vi "Get error details.vi"(8 "error in (no error)":errorcluster, 11 "JSONMessage in":refnum<class "WampMessage JSON.lvclass">) -> (0 "error out":errorcluster, 2 "Combined Error (JSON)":T1={"Error?"=FALSE, "WAMP Error"={"URI"="", "Arguments Payload"="", "ArgumentKw Payload"="{}", "Details"="{}", "Associated LabVIEW Error"={"status"=FALSE, "code"=0, "source"=""}}, "Associated LabVIEW Error"={"status"=FALSE, "code"=0, "source"=""}}, 3 "JSONMessage out":refnum<class "WampMessage JSON.lvclass">)   [LabVIEW 2020]
uses:
  WAMP Client/API/TypeDefs/Error or abort detail (JSON).ctl
  wamplv.lvlib
  <vilib>/Utility/error.llb/Error Cluster From Error Code.vi
  <vilib>/ErrorRing/Error Ring.xnode
  WampMessage JSON.lvclass
  WAMP Client/API/TypeDefs/Combined error.ctl
  Utils/Utils.lvclass
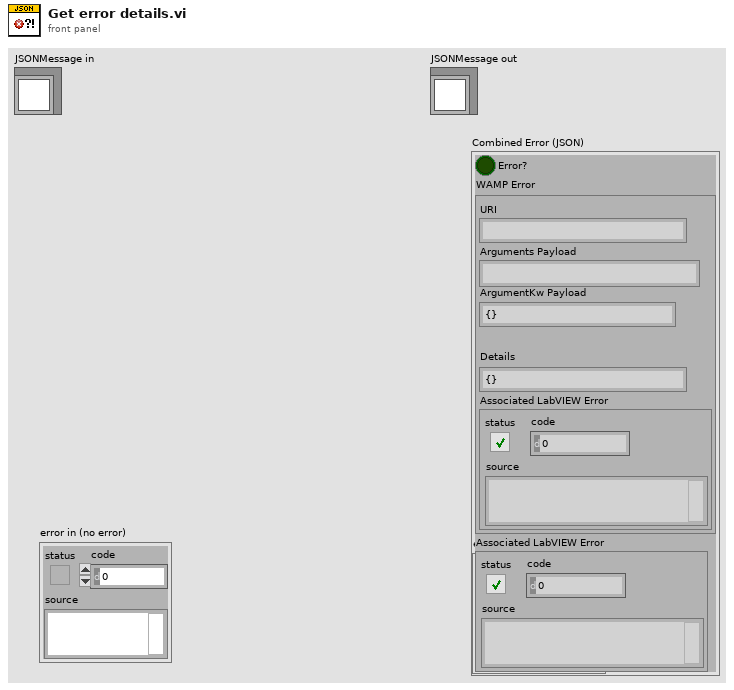
[diagram p1: front panel]
types:
  T1 = typedef "wamplv.lvlib/Combined error.ctl" = cluster{"Error?":bool, "WAMP Error":T2, "Associated LabVIEW Error":errorcluster}
  T2 = typedef "wamplv.lvlib/Error or abort detail (JSON).ctl" = cluster{"URI":string, "Arguments Payload":string, "ArgumentKw Payload":string, "Details":string, "Associated LabVIEW Error":errorcluster}
  T3 = typedef "wamplv.lvlib/WAMP Message Codes.ctl" = enum8{"HELLO", "WELCOME", "CHALLENGE", "AUTHENTICATE", "ABORT", "GOODBYE", "ERROR", "PUBLISH", "PUBLISHED", "SUBSCRIBE", "SUBSCRIBED", "UNSUBSCRIBE", "UNSUBSCRIBED", "EVENT", "CALL", "RESULT", "REGISTER", "REGISTERED", "UNREGISTER", "UNREGISTERED", "INVOCATION", "YIELD"}
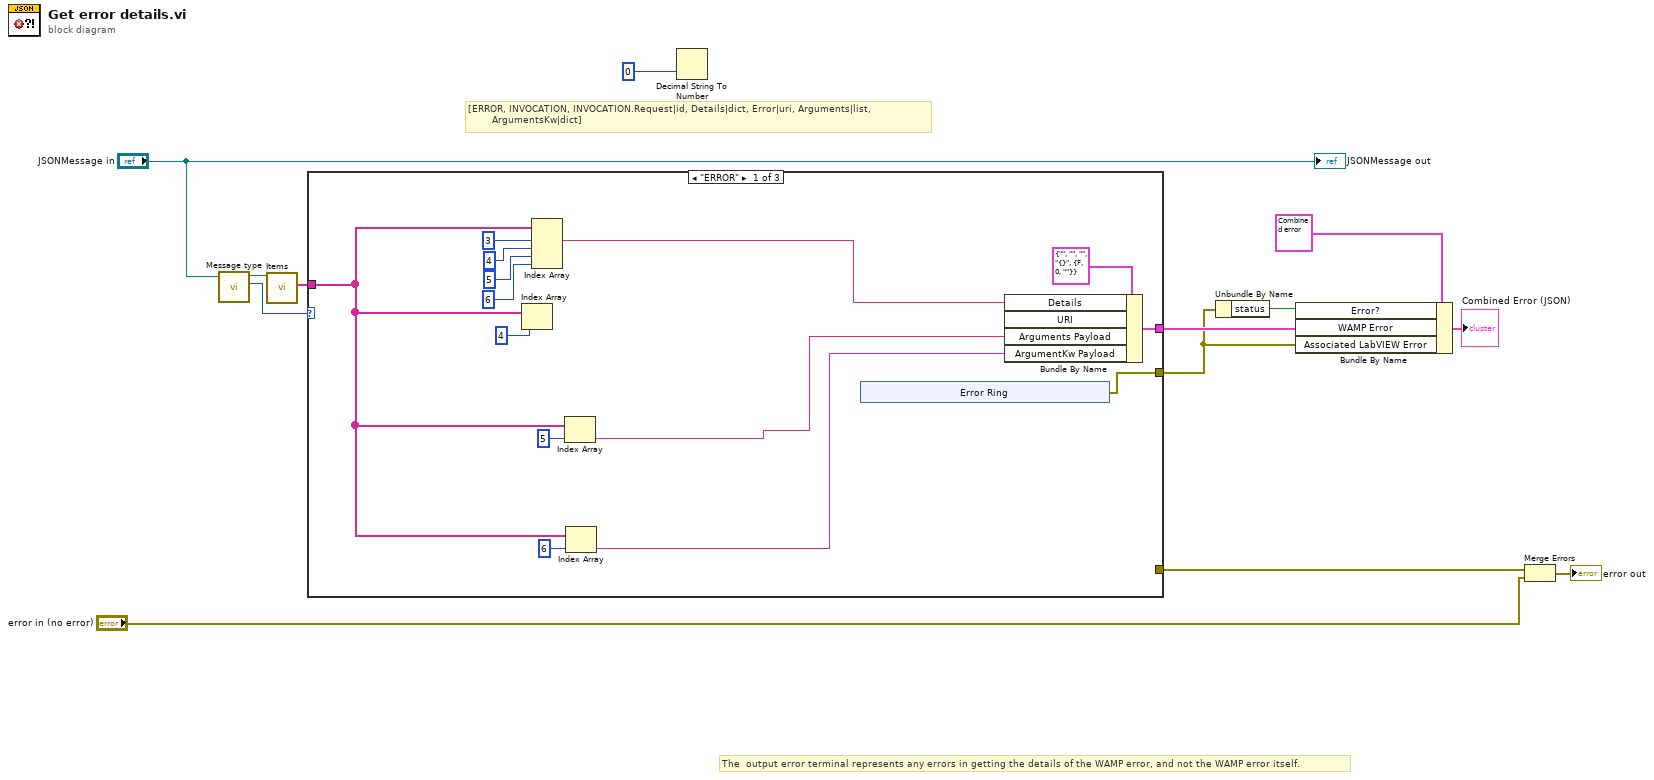
[diagram p0: block diagram]
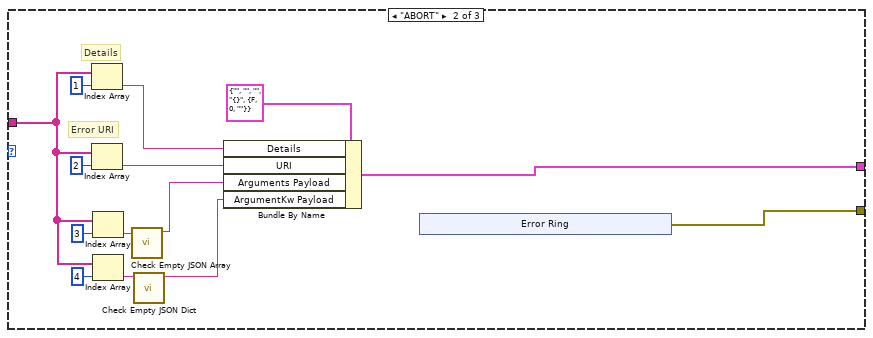
[diagram p2: hidden frame]
diagram:
  # "[ERROR, INVOCATION, INVOCATION.Request|id, Details|dict, Error|uri, Arguments|list,\n        ArgumentsKw|dict]"
  # "The  output error terminal represents any errors in getting the details of the WAMP error, and not the WAMP error itself."
  n1 = call-dynamic "Message type.vi"("JSONMessage in"="JSONMessage in") -> ("Message Codes"=w12:T3, "JSONMessage out"=w13:refnum<class "WampMessage JSON.lvclass">)  [unwired: 9 in]
  n2 = call-dynamic "Items.vi"("JSONMessage in"=w13) -> ("<JSON>Elements"=w11:string[])  [unwired: 9 in, 1 out]
  n3 = case shown="\"ERROR\"" w12 {
    tunnel: w11 -> [w28 w35 _]
    tunnel: [w23 w41 _] -> w7
    tunnel: [w24 w40 _] -> w8
    tunnel: [_ _ _] -> w6
    frame "ERROR" {
      # "ERROR"
      n4 = Index Array(array=w28, index=4) -> ()  [unwired: 1 out]
      n5 = Index Array(array=w28, index #1=3 ("index"), index #2=4 ("index"), index #3=5 ("index"), index #4=6 ("index")) -> (element #1=w21:string)  [unwired: 3 out]
      n6 = Index Array(array=w28, index=5) -> (element=w25:string)
      n7 = Index Array(array=w28, index=6) -> (element=w26:string)
      n8 = xnode "Error Ring"() -> ("error out"=w23:errorcluster)
      n9 = Bundle By Name(cluster=T2 {"URI"="", "Arguments Payload"="", "ArgumentKw Payload"="", "Details"="{}", "Associated LabVIEW Error"={"status"=FALSE, "code"=0, "source"=""}} ("Cluster"), "Details"=w21, "Arguments Payload"=w25, "ArgumentKw Payload"=w26) -> (w24:T2)  [unwired: 1 in]
    }
    frame "ABORT" {
      # "Details"
      # "Error URI"
      # "ABORT"
      n10 = Index Array(array=w35, index=1) -> (element=w44:string)
      n11 = Index Array(array=w35, index=2) -> (element=w45:string)
      n12 = Index Array(array=w35, index=3) -> (element=w37:string)
      n13 = Index Array(array=w35, index=4) -> (element=w36:string)
      n14 = call "Check Empty JSON Array.vi"("JSON in"=w37) -> ("JSON out"=w34:string)  [unwired: 10 in]
      n15 = call "Check Empty JSON Dict.vi"("JSON in"=w36) -> ("JSON out"=w33:string)  [unwired: 10 in]
      n16 = Bundle By Name(cluster=T2 {"URI"="", "Arguments Payload"="", "ArgumentKw Payload"="", "Details"="{}", "Associated LabVIEW Error"={"status"=FALSE, "code"=0, "source"=""}} ("Cluster"), "Details"=w44, "URI"=w45, "Arguments Payload"=w34, "ArgumentKw Payload"=w33) -> (w40:T2)
      n17 = xnode "Error Ring"() -> ("error out"=w41:errorcluster)
    }
    frame Default {
    }
  }
  n18 = Decimal String To Number(default (0L)=u64 0) -> (string=w2:string)  [unwired: 1 in, 2 out]
  n19 = Unbundle By Name(w7) -> ("status"=w9:bool)
  n20 = Bundle By Name(cluster=T1 {"Error?"=FALSE, "WAMP Error"={"URI"="", "Arguments Payload"="", "ArgumentKw Payload"="{}", "Details"="{}", "Associated LabVIEW Error"={"status"=FALSE, "code"=0, "source"=""}}, "Associated LabVIEW Error"={"status"=FALSE, "code"=0, "source"=""}} ("Combined Error"), "Error?"=w9, "WAMP Error"=w8, "Associated LabVIEW Error"=w7) -> (→"Combined Error (JSON)":T1)
  n21 = Merge Errors(w6, "error in (no error)") -> (→"error out":errorcluster)
  "JSONMessage out" <- "JSONMessage in"
